vi "Shot RPM Ready.vi"(10 "Current RPM":dbl, 11 "RPM Target":dbl) -> (0 "Shooter RPM Ready?":bool, 3 "RPM Out":dbl)   [LabVIEW 2016]
uses:
  Robot Global Data.vi
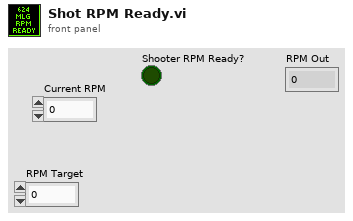
[diagram p1: front panel]
types:
  T1 = typedef "Dashboard Control Data.ctl" = cluster{"Drivetrain Settings":T2, "Intake Presets ":T4, "Shooter Presets":T5, "Vision Target Packet":T8, "Auton Presets":cluster{"Start Position":dbl}, "Drivetrain Encoder Values":T9, "Drivetrain Encoder Settings":cluster{"Left Tick Constant":dbl, "Right Tick Contant":dbl, "Reset Encoders":bool, "Center Tick Constant":dbl}, "Zero Gyro":bool}
  T2 = typedef "Drivetrain Settings.ctl" = cluster{"Gyro Tolerance":dbl, "Gyro Steer PID Gains":T3, "Y Power Multiplier":dbl, "Turn Power Multiplier":dbl, "Gyro Output":dbl, "Creep Rate":dbl, "Distance Drive PID Gains":T3, "Distance Tolerance":dbl, "Distance Output":dbl, "Strafe Threshold":dbl, "Strafe Correct":bool, "Strafe Corect Tolerance":dbl, "Translate Drive PID Gains":T3, "Strafe Output":dbl, "SC Right":dbl, "SC Left":dbl}
  T3 = typedef "PID Gains.ctl" = cluster{"proportional gain (Kc)":dbl, "integral time (Ti, min)":dbl, "derivative time (Td, min)":dbl}
  T4 = typedef "Intake Presets.ctl" = cluster{"Intake Speed ":dbl, "Outake Speed":dbl, "Current Trip Delay":dbl, "Max Current":dbl}
  T5 = typedef "Shooter Presets.ctl" = cluster{"Key Shot":cluster{"RPM ":dbl, "Hood?":bool}, "Distance Shot":cluster{"RPM":dbl, "Hood?":bool}, "RPM Tolerance":dbl, "Wheel C":dbl, "Vision Shot Presets":T6, "Hopper speed":dbl, "manuel presets":T7}
  T6 = typedef "Vision Shot Presets.ctl" = cluster{"Vision Dist RPM":dbl, "Vision RPM ":dbl, "Vision Dist Hood":bool, "Vision Hood":bool, "Vision Far Dist":dbl, "is we far??":bool}
  T7 = typedef "Manual Shooter Presets.ctl" = cluster{"change delay":dbl}
  T8 = typedef "Vision Target Packet.ctl" = cluster{"Robot Center":dbl, "Center X":dbl, "Center Y":dbl, "Angle":dbl, "Distance":dbl, "Found Target?":bool}
  T9 = typedef "Drivetrain Encoder Values.ctl" = cluster{"Left Encoder":T10, "Center Encoder":T10, "Right Encoder":T10}
  T10 = typedef "Encoder Values.ctl" = cluster{"Distance":dbl, "Speed":dbl, "Tick":dbl}
  T11 = typedef "Dashboard Display Data.ctl" = cluster{"Climb Status Cluster":T12, "Drivetrain Status Cluster":T13, "Intake Status Cluster":T14, "Shooter Status Cluster":T18, "Drivetrain Encoder Values":T9}
  T12 = typedef "Climb Status Cluster.ctl" = cluster{"Climb Speed":dbl}
  T13 = typedef "Drivetrain Status Cluster.ctl" = cluster{"Drivetrain Mode":enum16{"Manual", "Gyro Steer"}, "Y (Throttle)":dbl, "X (Steer)":dbl, "Z (Strafe)":dbl, "Heading Target":dbl, "Center Piston Down?":bool, "Traction?":bool, "Gyro Steer Finished?":bool, "Distance Drive Finished?":bool, "Gyro":dbl, "Distance Target":dbl, "Y Max Output":dbl, "Y Min Output":dbl, "X Max Output":dbl, "X Min Output":dbl, "Z Max Output":dbl, "Z Min Output":dbl, "Translation Target":dbl, "Translation Drive Finished?":bool}
  T14 = typedef "Intake Status Cluster.ctl" = cluster{"Roller Power":dbl, "Intake Mode":T15, "Intake Auto State":T16, "Backward Tripped?":bool, "Forward Tripped?":bool, "Filling Hopper?":bool, "Intake Current Trip State":T17, "Getting Gear?":bool}
  T15 = typedef "Intake Modes.ctl" = enum16{"Manual", "Auto"}
  T16 = typedef "Intake Auto States.ctl" = enum16{"Outake Ball", "Idle", "Load Ball"}
  T17 = typedef "Intake Trip States.ctl" = enum16{"Normal", "Backward Tripped", "Forward Tripped"}
  T18 = typedef "Shooter Status Cluster.ctl" = cluster{"RPM":dbl, "Shooter RPM Ready?":bool, "Hopper Speed":dbl, "Shooter Mode":T19, "Shot Type":T20, "Shooter State":T21}
  T19 = typedef "Shooter Modes.ctl" = enum16{"Auto", "Manual"}
  T20 = typedef "Shot Type.ctl" = enum16{"Dist Shot", "Key Shot"}
  T21 = typedef "Shooter Commands.ctl" = enum16{"Idle ", "Warmup ", "Shoot"}
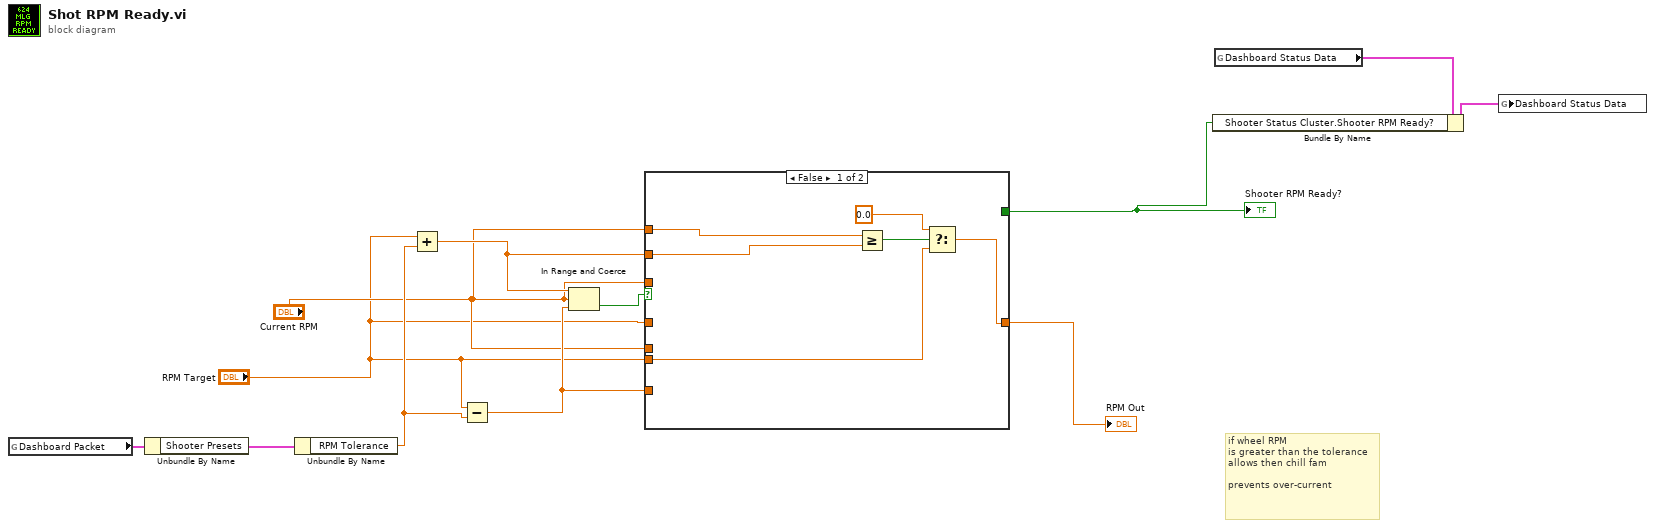
[diagram p0: block diagram]
diagram:
  # "if wheel RPM \nis greater than the tolerance \nallows then chill fam \n\nprevents over-current"
  n1 = global read "Robot Global Data.vi" "Dashboard Packet"() -> (w12:T1)
  n2 = Unbundle By Name(w12) -> ("Shooter Presets"=w11:T5)
  n3 = Unbundle By Name(w11) -> ("RPM Tolerance"=w8:dbl)
  n4 = Add(x="RPM Target", y=w8) -> (x+y=w5:dbl)
  n5 = Subtract(x="RPM Target", y=w8) -> (x-y=w4:dbl)
  n6 = In Range and Coerce(upper limit=w5, x="Current RPM", lower limit=w4) -> (In Range?=w7:bool)  [unwired: 1 out]
  n7 = case shown="False" w7 {
    selector: w7 -> [_ w20]
    tunnel: [_ w20] -> w3
    tunnel: "RPM Target" -> [_ w19]
    tunnel: [w14 w19] -> w6
    tunnel: "Current RPM" -> [w18 _]
    tunnel: w5 -> [w17 _]
    tunnel: "Current RPM" -> [_ _]
    tunnel: w4 -> [_ _]
    tunnel: "Current RPM" -> [_ _]
    tunnel: "RPM Target" -> [w13 _]
    frame False {
      n8 = Greater Or Equal?(x=w18, y=w17) -> (x >= y?=w16:bool)
      n9 = Select(t=0.0, s=w16, f=w13) -> (s? t:f=w14:dbl)
    }
    frame True {
    }
  }
  "Shooter RPM Ready?" <- w3
  "RPM Out" <- w6
  n10 = global read "Robot Global Data.vi" "Dashboard Status Data"() -> (w10:T11)
  n11 = Bundle By Name(cluster=w10, "Shooter Status Cluster.Shooter RPM Ready?"=w3) -> (w9:T11)
  n12 = global write "Robot Global Data.vi" "Dashboard Status Data"(w9) -> ()
